vi "Delimited String to Array_any delimiter.vi"(11 "Delimted String":string="a  b  c\rd\r\nf;g\nh,,i,,j") -> (3 "Array":string[](array[string]))   [LabVIEW 2023]
doc: "Divides string at any common delimiter: (one or more) space, new line, carraige return, comma, semicolon and returns array of strings.\n\nNote, two delimiters in a row will not produce an enpty array element."
uses:
  <vilib>/regexp/Match Regular Expression.xnode
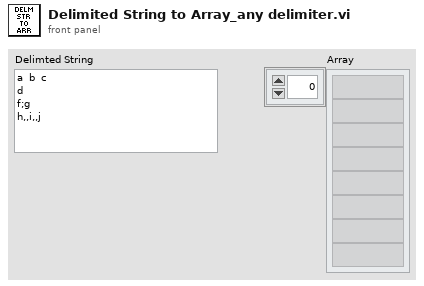
[diagram p1: front panel]
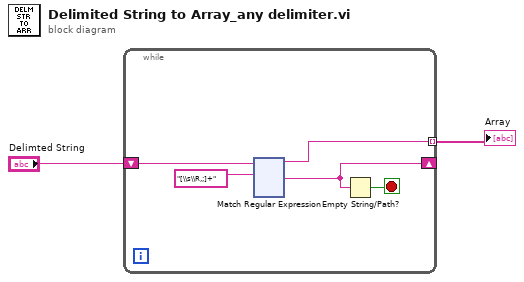
[diagram p0: block diagram]
diagram:
  n1 = while {
    shift-right: [w6] -> _
    shift-left: "Delimted String" -> [w7]
    tunnel: [w3] -> w1 mode=indexing
    stop <- w5 stop-if-true
    n2 = xnode "Match Regular Expression"("input string"=w7, "regular expression"="[\\s\\R,;]+") -> ("before match"=w3:string, "after match"=w6:string)  [unwired: 4 in, 3 out]
    n3 = Empty String/Path?(string/path=w6) -> (empty?=w5:bool)
  }
  "Array" <- w1
